vi "Set Ac Dc.vi"(10 "ac":i32, 11 "channel":u32) -> ()   [LabVIEW 2021, in "vmmso.lvlib"]
doc: "DLL_API void WINAPI SetAcDc(unsigned int channel, int ac);"
uses:
  vmmso.lvlib
  vmmso.dll
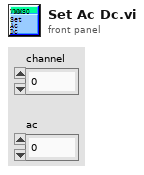
[diagram p1: front panel]
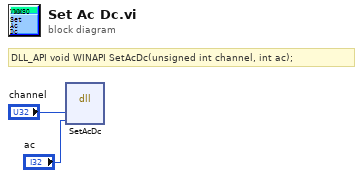
[diagram p0: block diagram]
diagram:
  # "DLL_API void WINAPI SetAcDc(unsigned int channel, int ac);"
  n1 = dll-call lib="D:/labviewdemo/LabviewDemo 21/vmmso/vmmso.*" fn="SetAcDc"("channel"="channel", "ac"="ac") -> ()  [unwired: 6 in, 2 out]
